vi "Main.vi"() -> ()   [LabVIEW 2020]
doc: "Use this template to build a simple state machine design pattern. Each state executes code and determines which state to transition to."
uses:
  State.ctl
  Data.ctl
panel:
  out "Ranking":cluster{"Score":dbl, "Login":string}[](array[cluster])
  in  "Close":bool
  in  "Add":bool
  in  "Login":string
  in  "Ranking":bool
  in  "Save":bool
  out "Colours":u32[](array[colorbox])
  in  "Exit":bool
  in  "Left":bool
  in  "Down":bool
  in  "Right":bool
  in  "Up":bool
  in  "Game Over":string="Game Over"
  in  "New Game":bool
  out "Score":i32
  in  "Board":i32[][](array[numeric])
  out "Buttons":refnum<vi>[][](array[refnum])
  in  "Button 9":bool caption="OK Button"
  in  "Button 16":bool caption="OK Button"
  in  "Button 15":bool caption="OK Button"
  in  "Button 14":bool caption="OK Button"
  in  "Button 13":bool caption="OK Button"
  in  "Button 12":bool caption="OK Button"
  in  "Button 11":bool caption="OK Button"
  in  "Button 10":bool caption="OK Button"
  in  "Button 8":bool caption="OK Button"
  in  "Button 7":bool caption="OK Button"
  in  "Button 6":bool caption="OK Button"
  in  "Button 5":bool caption="OK Button"
  in  "Button 4":bool caption="OK Button"
  in  "Button 3":bool caption="OK Button"
  in  "Button 2":bool caption="OK Button"
  in  "Button":bool caption="OK Button"
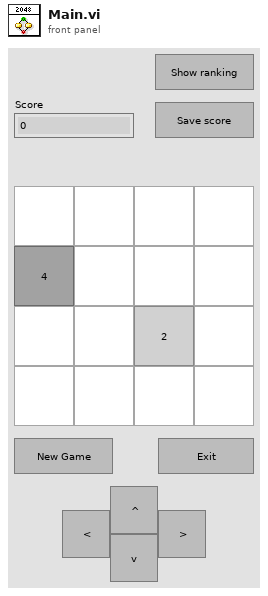
[diagram p1: front panel]
types:
  T1 = typedef "Data.ctl" = cluster{"Boolean <Replace Me>":bool, "String <Replace Me>":string, "Numeric <Replace Me>":dbl}
  T2 = typedef "State.ctl" = enum16{"INIT", "IDLE"}
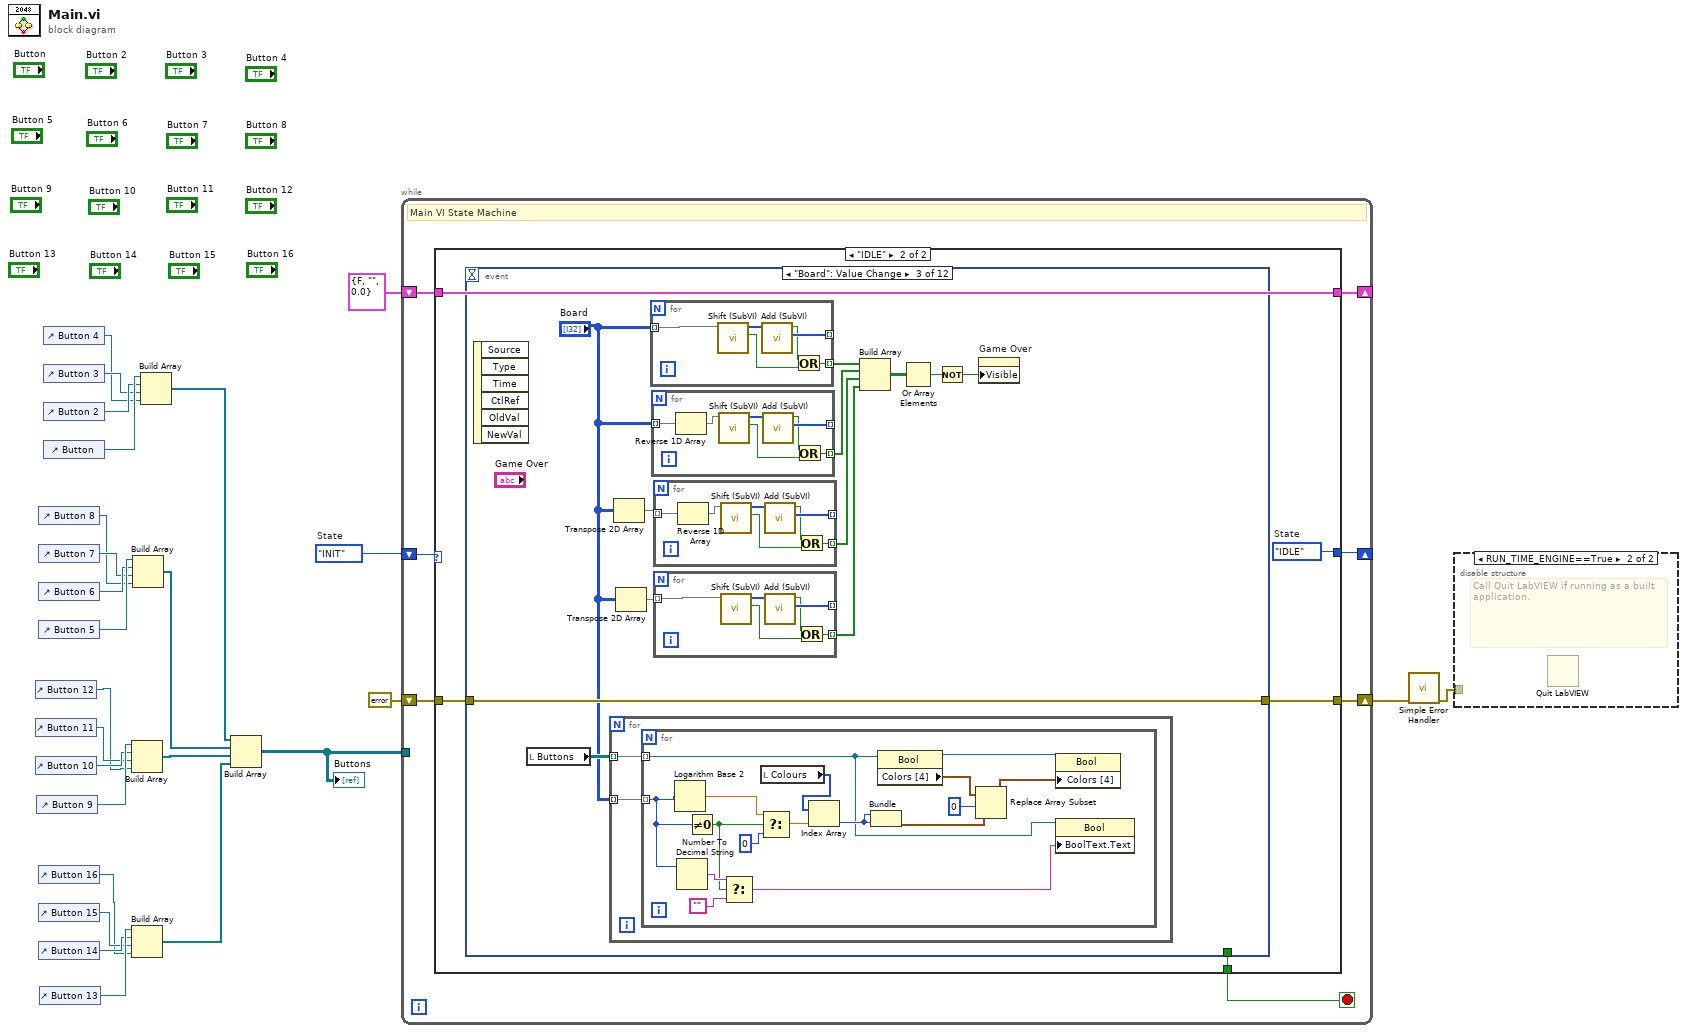
[diagram p0: block diagram]
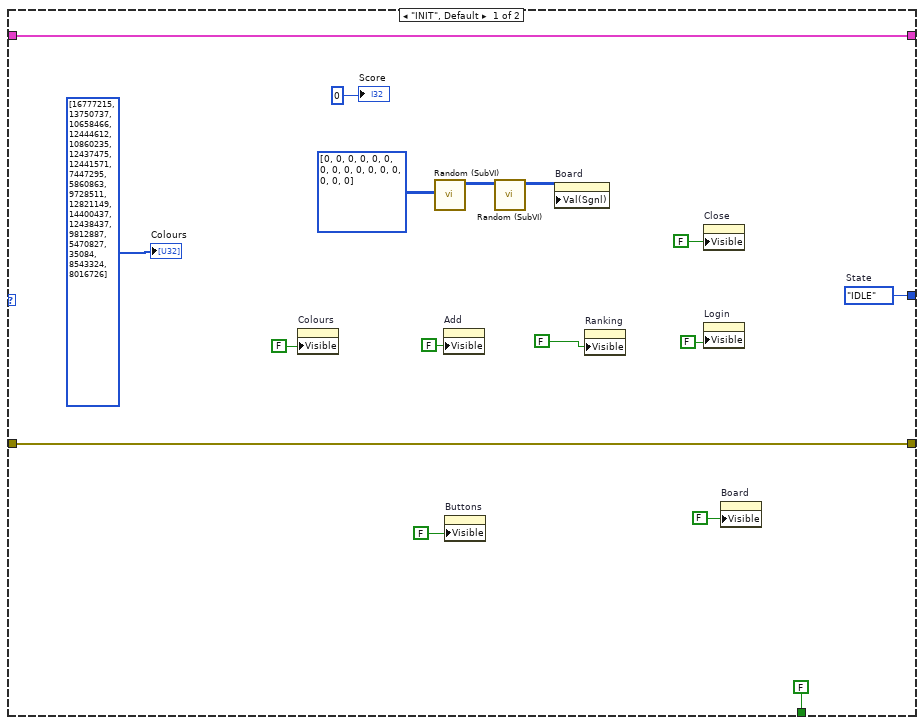
[diagram p3: hidden frame]
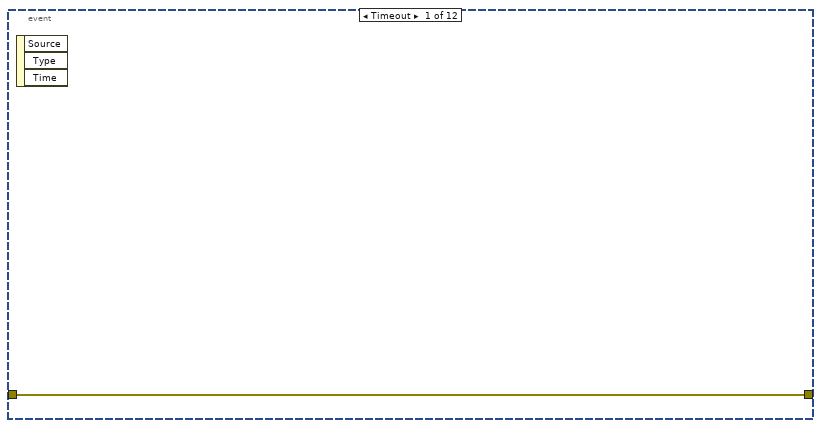
[diagram p4: hidden frame]
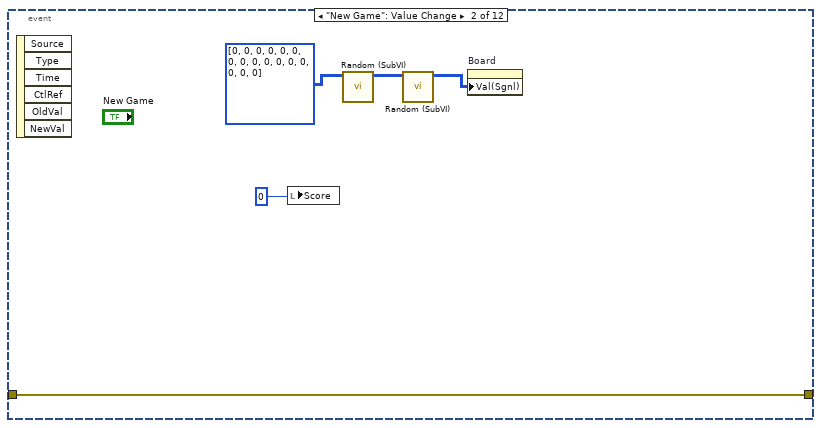
[diagram p5: hidden frame]
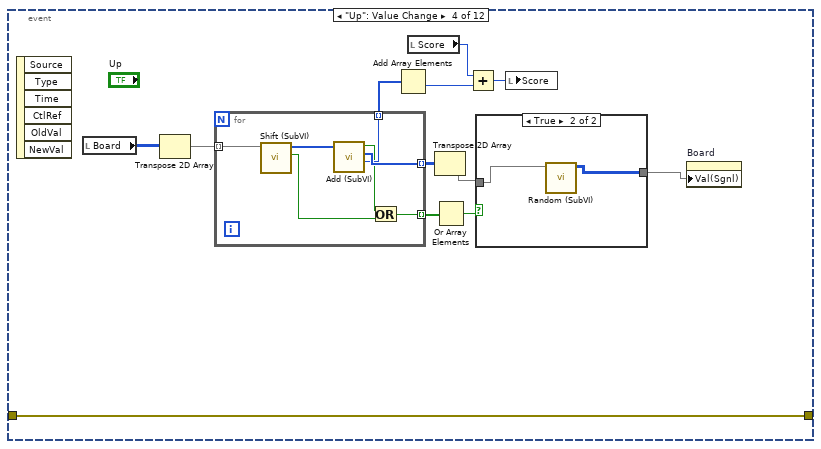
[diagram p6: hidden frame]
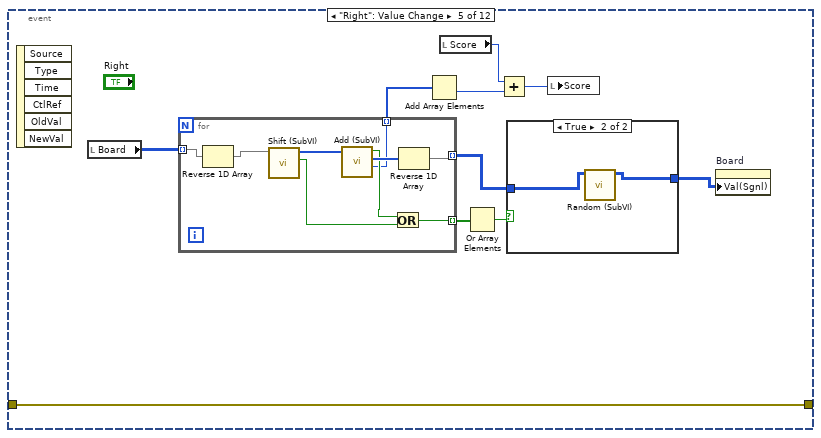
[diagram p8: hidden frame]
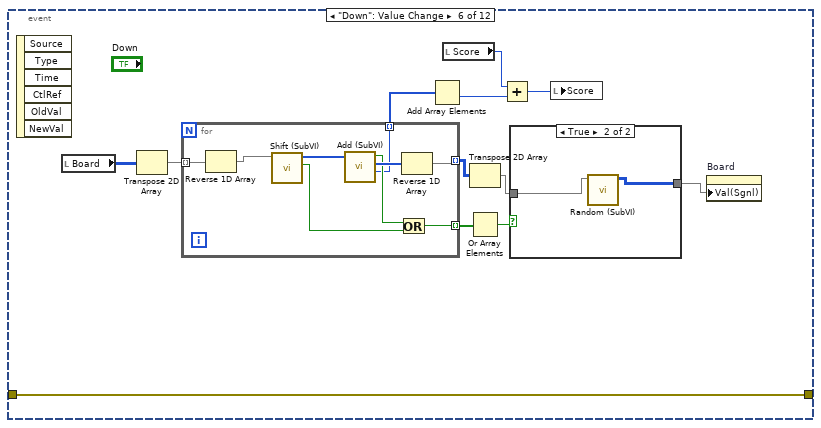
[diagram p10: hidden frame]
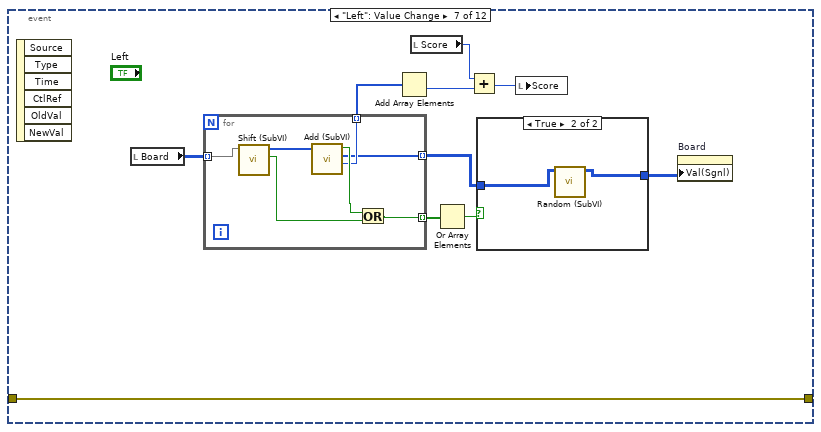
[diagram p12: hidden frame]
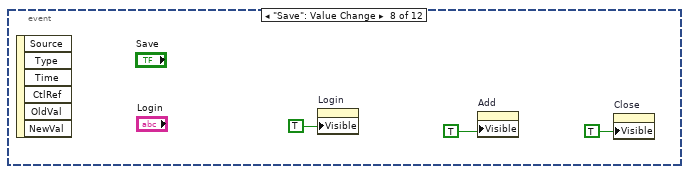
[diagram p14: hidden frame]
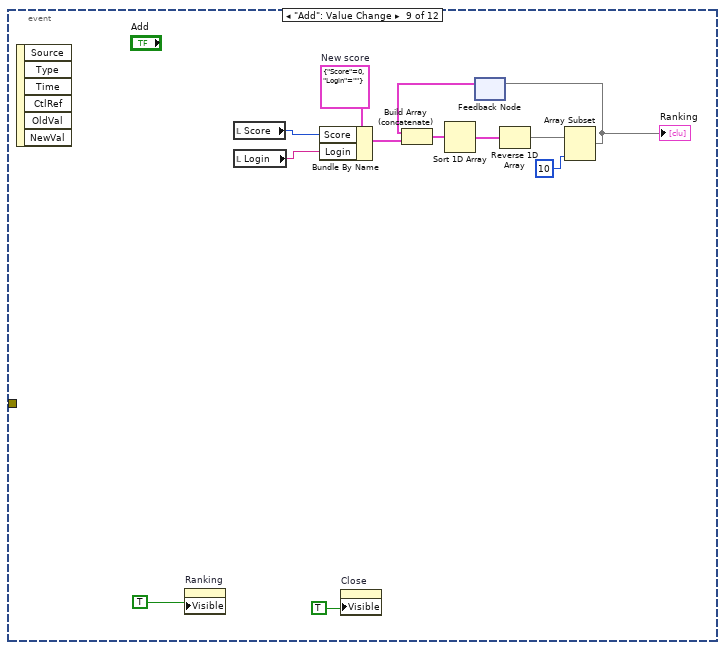
[diagram p15: hidden frame]
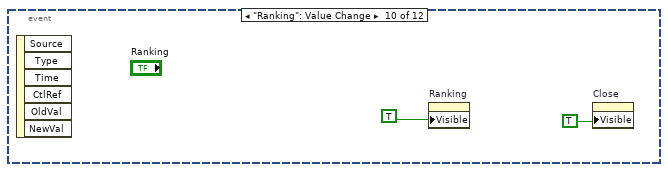
[diagram p16: hidden frame]
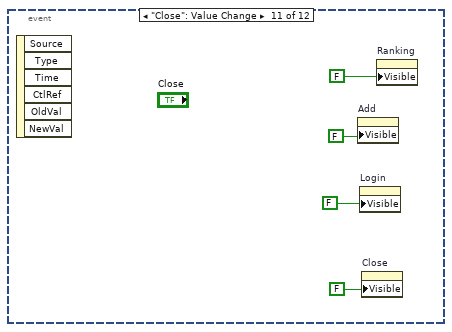
[diagram p17: hidden frame]
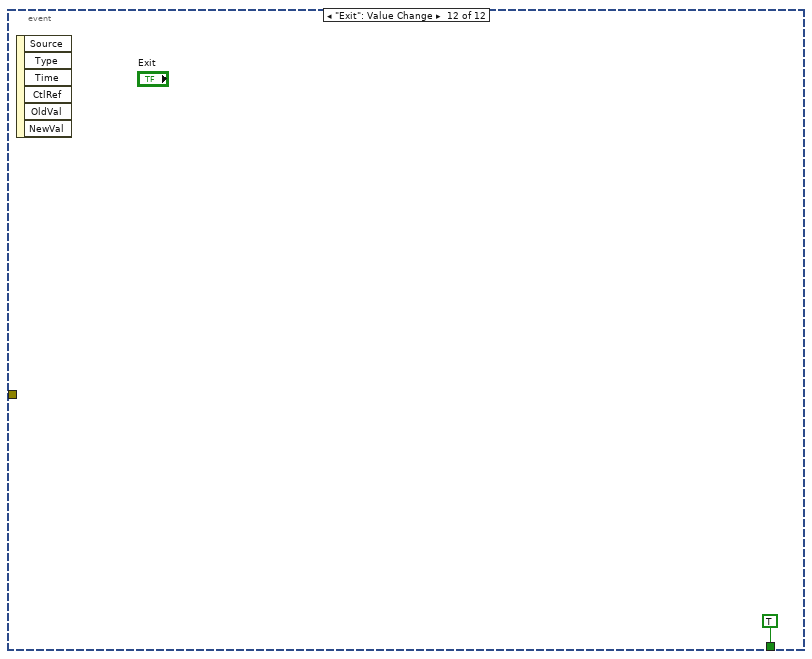
[diagram p18: hidden frame]
diagram:
  w26 = State."INIT"  # State
  n1 = control-ref of="Button 12"() -> (w10:refnum<vi>)
  n2 = control-ref of="Button 11"() -> (w11:refnum<vi>)
  n3 = control-ref of="Button 10"() -> (w12:refnum<vi>)
  n4 = control-ref of="Button 9"() -> (w13:refnum<vi>)
  n5 = control-ref of="Button 8"() -> (w14:refnum<vi>)
  n6 = control-ref of="Button 7"() -> (w15:refnum<vi>)
  n7 = control-ref of="Button 6"() -> (w16:refnum<vi>)
  n8 = control-ref of="Button 5"() -> (w17:refnum<vi>)
  n9 = control-ref of="Button 16"() -> (w6:refnum<vi>)
  n10 = control-ref of="Button 15"() -> (w7:refnum<vi>)
  n11 = control-ref of="Button 14"() -> (w8:refnum<vi>)
  n12 = control-ref of="Button 13"() -> (w9:refnum<vi>)
  n13 = control-ref of="Button 4"() -> (w18:refnum<vi>)
  n14 = control-ref of="Button 3"() -> (w19:refnum<vi>)
  n15 = control-ref of="Button 2"() -> (w20:refnum<vi>)
  n16 = control-ref of="Button"() -> (w21:refnum<vi>)
  n17 = Build Array(w13, w12, w11, w10) -> (w2:refnum<vi>[])
  n18 = Build Array(w9, w8, w7, w6) -> (w3:refnum<vi>[])
  n19 = Build Array(w17, w16, w15, w14) -> (w4:refnum<vi>[])
  n20 = Build Array(w21, w20, w19, w18) -> (w5:refnum<vi>[])
  n21 = Build Array(w5, w4, w2, w3) -> (w1:refnum<vi>[][])
  "Buttons" <- w1
  n22 = while {
    shift-right: [w32] -> _
    shift-left: w26 -> [w33]
    shift-right: [w29] -> _
    shift-left: T1 {"Boolean <Replace Me>"=FALSE, "String <Replace Me>"="", "Numeric <Replace Me>"=0.0} ("Data") -> [w28]
    shift-right: [w30] -> w23
    shift-left: errorcluster {"status"=FALSE, "code"=0, "source"=""} ("error constant") -> [w31]
    tunnel: w1 -> [_]
    stop <- w27 stop-if-true
    # "Main VI State Machine"
    n23 = case shown="\"IDLE\"" w33 {
      tunnel: [w46 w54] -> w32
      tunnel: w31 -> [w44 w53]
      tunnel: [w44 w52] -> w30
      tunnel: [w43 w51] -> w29
      tunnel: w28 -> [w43 w51]
      tunnel: [FALSE w50] -> w27
      frame "INIT", Default {
        w46 = State."IDLE"  # State
        n24 = property on="Colours" class="Arr (strict)"("Visible"=FALSE) -> ()  [unwired: 2 in, 2 out]
        n25 = call "Random (SubVI).vi"("Input"=i32[][] [[0, 0, 0, 0], [0, 0, 0, 0], [0, 0, 0, 0], [0, 0, 0, 0]]) -> ("Output"=w48:i32[][])  [unwired: 10 in]
        n26 = property on="Add" class="Bool"("Visible"=FALSE) -> ()  [unwired: 2 in, 2 out]
        n27 = property on="Buttons" class="Arr (strict)"("Visible"=FALSE) -> ()  [unwired: 2 in, 2 out]
        n28 = call "Random (SubVI).vi"("Input"=w48) -> ("Output"=w47:i32[][])  [unwired: 10 in]
        n29 = property on="Board" class="Arr (strict)"("Val(Sgnl)"=w47) -> ()  [unwired: 2 in, 2 out]
        n30 = property on="Ranking" class="Arr (strict)"("Visible"=FALSE) -> ()  [unwired: 2 in, 2 out]
        n31 = property on="Close" class="Bool"("Visible"=FALSE) -> ()  [unwired: 2 in, 2 out]
        n32 = property on="Login" class="Str"("Visible"=FALSE) -> ()  [unwired: 2 in, 2 out]
        n33 = property on="Board" class="Arr (strict)"("Visible"=FALSE) -> ()  [unwired: 2 in, 2 out]
        "Score" <- 0
        "Colours" <- u32[] [16777215, 13750737, 10658466, 12444612, 10860235, 12437475, 12441571, 7447295, 5860863, 9728511, 12821149, 14400437, 12438437, 9812887, 5470827, 35084, 8543324, 8016726]
      }
      frame "IDLE" {
        w54 = State."IDLE"  # State
        n34 = event shown="[2] \"Board\": Value Change" {
          selector: _ -> [_ _ _ _ _ _ _ _ _ _ _ _]
          dyn-events: _ -> [_ _ _ _ _ _ _ _ _ _ _ _]
          timeout: _ -> [_ _ _ _ _ _ _ _ _ _ _ _]
          tunnel: w53 -> [w55 w56 w72 w117 w139 w161 w185 _ _ _ _ _]
          tunnel: [w55 w56 w72 w117 w139 w161 w185 _ _ _ _ _] -> w52
          tunnel: [_ _ _ _ _ _ _ _ _ _ _ TRUE] -> w50
          event Timeout {
            n35 = event-data() -> ()  [unwired: 1 in, 3 out]
          }
          event "New Game": Value Change {
            n36 = event-data() -> ()  [unwired: 1 in, 6 out]
            n37 = local write "Score"(0) -> ()
            n38 = call "Random (SubVI).vi"("Input"=i32[][] [[0, 0, 0, 0], [0, 0, 0, 0], [0, 0, 0, 0], [0, 0, 0, 0]]) -> ("Output"=w60:i32[][])  [unwired: 10 in]
            n39 = call "Random (SubVI).vi"("Input"=w60) -> ("Output"=w59:i32[][])  [unwired: 10 in]
            n40 = property on="Board" class="Arr (strict)"("Val(Sgnl)"=w59) -> ()  [unwired: 2 in, 2 out]
          }
          event "Board": Value Change {
            n41 = event-data() -> ()  [unwired: 1 in, 6 out]
            n42 = local read "Buttons"() -> (w62:refnum<vi>[][])
            n43 = for {
              tunnel: "Board" -> [w74] mode=indexing
              tunnel: w62 -> [w73] mode=indexing
              n44 = for {
                tunnel: w74 -> [w76] mode=indexing
                tunnel: w73 -> [w78] mode=indexing
                n45 = Logarithm Base 2(1:w76) -> (0:w77:dbl)
                n46 = Number To Decimal String(number=w76) -> (decimal integer string=w90:string)  [unwired: 1 in]
                n47 = Not Equal To 0?(x=w76) -> (x != 0?=w88:bool)
                n48 = Select(t=w90, s=w88, f="") -> (s? t:f=w79:string)
                n49 = local read "Colours"() -> (w75:u32[])
                n50 = Select(t=w77, s=w88, f=0) -> (s? t:f=w86:dbl)
                n51 = Index Array(array=w75, index=w86) -> (element=w85:u32)
                n52 = Bundle("Color Box"=w85, "Color Box"=w85) -> (w82:cluster{"Color Box":u32, "Color Box":u32})  [unwired: 1 in]
                n53 = property class="Bool"(reference=w78) -> (reference out=w81:refnum<vi>, "Colors [4]"=w83:cluster{u32, u32}[])  [unwired: 1 in, 1 out]
                n54 = Replace Array Subset(array=w83, new element=w82, index=0) -> (w80:cluster{u32, u32}[])
                n55 = property class="Bool"(reference=w81, "Colors [4]"=w80) -> ()  [unwired: 1 in, 2 out]
                n56 = property class="Bool"(reference=w78, "BoolText.Text"=w79) -> ()  [unwired: 1 in, 2 out]
              }
            }
            n57 = Transpose 2D Array(2D array="Board") -> (transposed array=w70:i32[][])
            n58 = Transpose 2D Array(2D array="Board") -> (transposed array=w71:i32[][])
            n59 = for {
              tunnel: "Board" -> [w115] mode=indexing
              tunnel: [w116] -> w67 mode=indexing
              tunnel: [w113] -> _ mode=indexing
              n60 = call "Shift (SubVI).vi"("Input Shift"=w115) -> ("Shift changed?"=w111:bool, "Output Shift"=w114:i32[])  [unwired: 9 in]
              n61 = call "Add (SubVI).vi"("Input Add"=w114) -> ("Output Add 2"=w113:i32[], "Add changed?"=w112:bool)  [unwired: 8 in, 1 out]
              n62 = Or(x=w112, y=w111) -> (x .or. y?=w116:bool)
            }
            n63 = for {
              tunnel: [w104] -> w64 mode=indexing
              tunnel: [w102] -> _ mode=indexing
              tunnel: "Board" -> [w98] mode=indexing
              n64 = Reverse 1D Array(array=w98) -> (reversed array=w99:i32[])
              n65 = call "Shift (SubVI).vi"("Input Shift"=w99) -> ("Shift changed?"=w100:bool, "Output Shift"=w103:i32[])  [unwired: 9 in]
              n66 = call "Add (SubVI).vi"("Input Add"=w103) -> ("Output Add 2"=w102:i32[], "Add changed?"=w101:bool)  [unwired: 8 in, 1 out]
              n67 = Or(x=w101, y=w100) -> (x .or. y?=w104:bool)
            }
            n68 = for {
              tunnel: [w97] -> w65 mode=indexing
              tunnel: [w95] -> _ mode=indexing
              tunnel: w70 -> [w91] mode=indexing
              n69 = Reverse 1D Array(array=w91) -> (reversed array=w92:i32[])
              n70 = call "Shift (SubVI).vi"("Input Shift"=w92) -> ("Shift changed?"=w93:bool, "Output Shift"=w96:i32[])  [unwired: 9 in]
              n71 = call "Add (SubVI).vi"("Input Add"=w96) -> ("Output Add 2"=w95:i32[], "Add changed?"=w94:bool)  [unwired: 8 in, 1 out]
              n72 = Or(x=w94, y=w93) -> (x .or. y?=w97:bool)
            }
            n73 = for {
              tunnel: w71 -> [w109] mode=indexing
              tunnel: [w110] -> w66 mode=indexing
              tunnel: [w107] -> _ mode=indexing
              n74 = call "Shift (SubVI).vi"("Input Shift"=w109) -> ("Shift changed?"=w105:bool, "Output Shift"=w108:i32[])  [unwired: 9 in]
              n75 = call "Add (SubVI).vi"("Input Add"=w108) -> ("Output Add 2"=w107:i32[], "Add changed?"=w106:bool)  [unwired: 8 in, 1 out]
              n76 = Or(x=w106, y=w105) -> (x .or. y?=w110:bool)
            }
            n77 = Build Array(w67, w64, w65, w66) -> (w68:bool[][])
            n78 = Or Array Elements(Boolean array=w68) -> (logical OR=w69:bool)
            n79 = Not(x=w69) -> (.not. x?=w63:bool)
            n80 = property on="Game Over" class="Str"("Visible"=w63) -> ()  [unwired: 2 in, 2 out]
          }
          event "Up": Value Change {
            n81 = event-data() -> ()  [unwired: 1 in, 6 out]
            n82 = local read "Board"() -> (w123:i32[][])
            n83 = Transpose 2D Array(2D array=w123) -> (transposed array=w125:i32[][])
            n84 = for {
              tunnel: w125 -> [w137] mode=indexing
              tunnel: [w138] -> w127 mode=indexing
              tunnel: [w135] -> w122 mode=indexing
              tunnel: [w134] -> w121 mode=indexing
              n85 = call "Shift (SubVI).vi"("Input Shift"=w137) -> ("Shift changed?"=w132:bool, "Output Shift"=w136:i32[])  [unwired: 9 in]
              n86 = call "Add (SubVI).vi"("Input Add"=w136) -> ("Score 2"=w134:i32, "Output Add 2"=w135:i32[], "Add changed?"=w133:bool)  [unwired: 8 in]
              n87 = Or(x=w133, y=w132) -> (x .or. y?=w138:bool)
            }
            n88 = Add Array Elements(numeric array=w121) -> (sum=w128:i32)
            n89 = local read "Score"() -> (w120:i32)
            n90 = Transpose 2D Array(2D array=w122) -> (transposed array=w124:i32[][])
            n91 = Or Array Elements(Boolean array=w127) -> (logical OR=w126:bool)
            n92 = Add(x=w120, y=w128) -> (x+y=w119:i32)
            n93 = case shown="True" w126 {
              tunnel: w124 -> [w129 w131]
              tunnel: [w129 w130] -> w118
              frame False {
              }
              frame True {
                n94 = call "Random (SubVI).vi"("Input"=w131) -> ("Output"=w130:i32[][])  [unwired: 10 in]
              }
            }
            n95 = local write "Score"(w119) -> ()
            n96 = property on="Board" class="Arr (strict)"("Val(Sgnl)"=w118) -> ()  [unwired: 2 in, 2 out]
          }
          event "Right": Value Change {
            n97 = event-data() -> ()  [unwired: 1 in, 6 out]
            n98 = local read "Board"() -> (w143:i32[][])
            n99 = for {
              tunnel: [w160] -> w146 mode=indexing
              tunnel: [w159] -> w147 mode=indexing
              tunnel: w143 -> [w155] mode=indexing
              tunnel: [w153] -> w142 mode=indexing
              n100 = Reverse 1D Array(array=w155) -> (reversed array=w156:i32[])
              n101 = call "Shift (SubVI).vi"("Input Shift"=w156) -> ("Shift changed?"=w152:bool, "Output Shift"=w157:i32[])  [unwired: 9 in]
              n102 = call "Add (SubVI).vi"("Input Add"=w157) -> ("Score 2"=w153:i32, "Output Add 2"=w158:i32[], "Add changed?"=w154:bool)  [unwired: 8 in]
              n103 = Or(x=w154, y=w152) -> (x .or. y?=w160:bool)
              n104 = Reverse 1D Array(array=w158) -> (reversed array=w159:i32[])
            }
            n105 = Add Array Elements(numeric array=w142) -> (sum=w148:i32)
            n106 = local read "Score"() -> (w141:i32)
            n107 = Or Array Elements(Boolean array=w146) -> (logical OR=w145:bool)
            n108 = Add(x=w141, y=w148) -> (x+y=w140:i32)
            n109 = case shown="True" w145 {
              tunnel: w147 -> [w149 w150]
              tunnel: [w149 w151] -> w144
              frame False {
              }
              frame True {
                n110 = call "Random (SubVI).vi"("Input"=w150) -> ("Output"=w151:i32[][])  [unwired: 10 in]
              }
            }
            n111 = local write "Score"(w140) -> ()
            n112 = property on="Board" class="Arr (strict)"("Val(Sgnl)"=w144) -> ()  [unwired: 2 in, 2 out]
          }
          event "Down": Value Change {
            n113 = event-data() -> ()  [unwired: 1 in, 6 out]
            n114 = local read "Board"() -> (w166:i32[][])
            n115 = Transpose 2D Array(2D array=w166) -> (transposed array=w165:i32[][])
            n116 = for {
              tunnel: [w184] -> w171 mode=indexing
              tunnel: [w183] -> w167 mode=indexing
              tunnel: [w179] -> w169 mode=indexing
              tunnel: w165 -> [w178] mode=indexing
              n117 = Reverse 1D Array(array=w178) -> (reversed array=w177:i32[])
              n118 = call "Shift (SubVI).vi"("Input Shift"=w177) -> ("Shift changed?"=w176:bool, "Output Shift"=w181:i32[])  [unwired: 9 in]
              n119 = call "Add (SubVI).vi"("Input Add"=w181) -> ("Score 2"=w179:i32, "Output Add 2"=w182:i32[], "Add changed?"=w180:bool)  [unwired: 8 in]
              n120 = Or(x=w180, y=w176) -> (x .or. y?=w184:bool)
              n121 = Reverse 1D Array(array=w182) -> (reversed array=w183:i32[])
            }
            n122 = Add Array Elements(numeric array=w169) -> (sum=w172:i32)
            n123 = local read "Score"() -> (w164:i32)
            n124 = Transpose 2D Array(2D array=w167) -> (transposed array=w168:i32[][])
            n125 = Or Array Elements(Boolean array=w171) -> (logical OR=w170:bool)
            n126 = Add(x=w164, y=w172) -> (x+y=w163:i32)
            n127 = case shown="True" w170 {
              tunnel: w168 -> [w173 w174]
              tunnel: [w173 w175] -> w162
              frame False {
              }
              frame True {
                n128 = call "Random (SubVI).vi"("Input"=w174) -> ("Output"=w175:i32[][])  [unwired: 10 in]
              }
            }
            n129 = local write "Score"(w163) -> ()
            n130 = property on="Board" class="Arr (strict)"("Val(Sgnl)"=w162) -> ()  [unwired: 2 in, 2 out]
          }
          event "Left": Value Change {
            n131 = event-data() -> ()  [unwired: 1 in, 6 out]
            n132 = local read "Board"() -> (w189:i32[][])
            n133 = for {
              tunnel: [w204] -> w193 mode=indexing
              tunnel: [w201] -> w191 mode=indexing
              tunnel: [w199] -> w190 mode=indexing
              tunnel: w189 -> [w198] mode=indexing
              n134 = call "Shift (SubVI).vi"("Input Shift"=w198) -> ("Shift changed?"=w200:bool, "Output Shift"=w203:i32[])  [unwired: 9 in]
              n135 = call "Add (SubVI).vi"("Input Add"=w203) -> ("Score 2"=w201:i32, "Output Add 2"=w199:i32[], "Add changed?"=w202:bool)  [unwired: 8 in]
              n136 = Or(x=w202, y=w200) -> (x .or. y?=w204:bool)
            }
            n137 = Add Array Elements(numeric array=w191) -> (sum=w194:i32)
            n138 = local read "Score"() -> (w187:i32)
            n139 = Or Array Elements(Boolean array=w193) -> (logical OR=w192:bool)
            n140 = Add(x=w187, y=w194) -> (x+y=w188:i32)
            n141 = case shown="True" w192 {
              tunnel: w190 -> [w195 w196]
              tunnel: [w195 w197] -> w186
              frame False {
              }
              frame True {
                n142 = call "Random (SubVI).vi"("Input"=w196) -> ("Output"=w197:i32[][])  [unwired: 10 in]
              }
            }
            n143 = local write "Score"(w188) -> ()
            n144 = property on="Board" class="Arr (strict)"("Val(Sgnl)"=w186) -> ()  [unwired: 2 in, 2 out]
          }
          event "Save": Value Change {
            n145 = event-data() -> ()  [unwired: 1 in, 6 out]
            n146 = property on="Login" class="Str"("Visible"=TRUE) -> ()  [unwired: 2 in, 2 out]
            n147 = property on="Add" class="Bool"("Visible"=TRUE) -> ()  [unwired: 2 in, 2 out]
            n148 = property on="Close" class="Bool"("Visible"=TRUE) -> ()  [unwired: 2 in, 2 out]
          }
          event "Add": Value Change {
            w217 = cluster{"Score":i32, "Login":string} {"Score"=0, "Login"=""}  # New score
            n149 = event-data() -> ()  [unwired: 1 in, 6 out]
            n150 = property on="Ranking" class="Arr (strict)"("Visible"=TRUE) -> ()  [unwired: 2 in, 2 out]
            n151 = local read "Score"() -> (w211:i32)
            n152 = local read "Login"() -> (w210:string)
            n153 = Bundle By Name(cluster=w217, "Score"=w211, "Login"=w210) -> (w218:cluster{"Score":i32, "Login":string})
            n154 = property on="Close" class="Bool"("Visible"=TRUE) -> ()  [unwired: 2 in, 2 out]
            n155 = feedback #1() -> (w213:cluster{"Score":i32, "Login":string}[])  [unwired: 1 in]
            n156 = Build Array (concatenate)(w213, w218) -> (w216:cluster{"Score":i32, "Login":string}[])
            n157 = Sort 1D Array(array=w216) -> (sorted array=w215:cluster{"Score":i32, "Login":string}[])
            n158 = Reverse 1D Array(array=w215) -> (reversed array=w214:cluster{"Score":i32, "Login":string}[])
            n159 = Array Subset(array=w214, length=10 ("Länge")) -> (w208:cluster{"Score":i32, "Login":string}[])  [unwired: 1 in]
            "Ranking" <- w208
            n160 = feedback-in #1(w208) -> ()
          }
          event "Ranking": Value Change {
            n161 = event-data() -> ()  [unwired: 1 in, 6 out]
            n162 = property on="Ranking" class="Arr (strict)"("Visible"=TRUE) -> ()  [unwired: 2 in, 2 out]
            n163 = property on="Close" class="Bool"("Visible"=TRUE) -> ()  [unwired: 2 in, 2 out]
          }
          event "Close": Value Change {
            n164 = event-data() -> ()  [unwired: 1 in, 6 out]
            n165 = property on="Add" class="Bool"("Visible"=FALSE) -> ()  [unwired: 2 in, 2 out]
            n166 = property on="Login" class="Str"("Visible"=FALSE) -> ()  [unwired: 2 in, 2 out]
            n167 = property on="Close" class="Bool"("Visible"=FALSE) -> ()  [unwired: 2 in, 2 out]
            n168 = property on="Ranking" class="Arr (strict)"("Visible"=FALSE) -> ()  [unwired: 2 in, 2 out]
          }
          event "Exit": Value Change {
            n169 = event-data() -> ()  [unwired: 1 in, 6 out]
          }
        }
      }
    }
  }
  n170 = call <vilib>:"Simple Error Handler.vi"("error in (no error)"=w23) -> ("error out"=w22:errorcluster)  [unwired: 4 in, 4 out]
  n171 = disable-structure shown="RUN_TIME_ENGINE==True" {
    disable-tunnel: w22 -> [_ _]
    frame condition #0 (active) {
    }
    frame condition #1 {
      # "Call Quit LabVIEW if running as a built application."
      n172 = Quit LabVIEW() -> ()  [unwired: 1 in]
    }
  }
